vi "Begin.vi"(8 "error in":errorcluster) -> (0 "error out":errorcluster)   [LabVIEW 2019]
doc: "Called before other user functions, this VI is expected to open initial I/O refnums, load in file data, and do all program initialization. Notice that the <B>error out</B> terminal is simply used for data flow. Wiring it to other structures or subVIs ensures that this VI runs first."
uses:
  <vilib>/Rock Robotics/WPI/DriverStation/WPI_DriverStationRobotMode2.ctl
  <vilib>/Rock Robotics/WPI/Joystick/WPI_JoystickDeviceEnum.ctl
  <vilib>/Rock Robotics/WPI/SafetyOutput/WPI_SafetyOutputConfigMenu.ctl
  <vilib>/Rock Robotics/WPI/ThirdParty/Phoenix-LabVIEW/Motor Controller/Controls/CTRE_Phoenix_MotorControl_NeutralMode.ctl
  <vilib>/Rock Robotics/WPI/ThirdParty/Phoenix-LabVIEW/Motor Controller/Controls/CTRE_Phoenix_MotorControl_StatorCurrentLimitConfiguration.ctl
  <vilib>/Rock Robotics/WPI/ThirdParty/Phoenix-LabVIEW/CANCoder/Controls/CTRE_Phoenix_CANcoder_SensorInitializationStrategy.ctl
  <vilib>/Rock Robotics/WPI/ThirdParty/Phoenix-LabVIEW/Motor Controller/Controls/CTRE_Phoenix_MotorControl_FeedbackDevice.ctl
  <vilib>/Rock Robotics/SystemInterfaces/DIO/FPGA_DIOPWMChannel.ctl
  <vilib>/Rock Robotics/WPI/Solenoid/WPI_SolenoidChannel.ctl
  <vilib>/Rock Robotics/SystemInterfaces/DIO/FPGA_DIOChannel.ctl
  Robot Global Data.vi
  <vilib>/Rock Robotics/Network Tables/NT Write String Array.vi
  Refnums.vi
  CAN.vi
  PID.vi
  <vilib>/Rock Robotics/WPI/ThirdParty/Phoenix-LabVIEW/Motor Controller/Sensor/CTRE_Phoenix_MotorControl_SetIntegratedSensorPosition_TalonFX.vi
  <vilib>/Rock Robotics/WPI/RobotDrive/WPI_RobotDriveOpen2MotorWithExistingMotors.vi
  <vilib>/Rock Robotics/WPI/MotorControl/WPI_MotorControlOpen SPARK.vi
  <vilib>/Rock Robotics/WPI/Utilities/WPI_GetSetVariantRefNum.vi
  <vilib>/Rock Robotics/WPI/Solenoid/WPI_SolenoidOpenDouble.vi
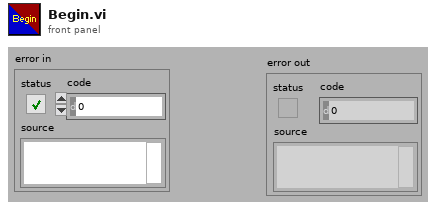
[diagram p1: front panel]
types:
  T1 = typedef "WPI_DriverStationRobotMode2.ctl" = enum16{"Autonomous Disabled", "Autonomous Enabled", "Teleop Disabled", "Teleop Enabled", "Disconnected", "Finish", "Test Disabled", "Test Enabled", "Emergency Stopped"}
  T2 = typedef "WPI_JoystickDeviceEnum.ctl" = enum16{"USB 0", "USB 1", "USB 2", "USB 3", "USB 4", "USB 5"}
  T3 = enum16{"FollowerType_PercentOutput", "FollowerType_AuxOutput1"}
  T4 = typedef "CTRE_Phoenix_CANcoder_SensorInitializationStrategy.ctl" = enum16{"Boot To Zero", "Boot To Absolute Position"}
  T5 = typedef "CTRE_Phoenix_MotorControl_StatorCurrentLimitConfiguration.ctl" = cluster{"Enable?":bool, "Current Limit":dbl, "Threshold Current":dbl, "Threshold Time":dbl}
  T6 = typedef "CTRE_Phoenix_MotorControl_NeutralMode.ctl" = enum8{"EEPROMSetting", "Override to Coast", "Override to Brake"}
  T7 = typedef "WPI_SafetyOutputConfigMenu.ctl" = enum16{"Enable", "Disable"}
  T8 = typedef "FPGA_DIOPWMChannel.ctl" = enum8{"PWM 0", "PWM 1", "PWM 2", "PWM 3", "PWM 4", "PWM 5", "PWM 6", "PWM 7", "PWM 8", "PWM 9", "PWM MXP 0", "PWM MXP 1", "PWM MXP 2", "PWM MXP 3", "PWM MXP 4", "PWM MXP 5", "PWM MXP 6", "PWM MXP 7", "PWM MXP 8", "PWM MXP 9", "Invalid"}
  T9 = enum16{"Blue + Yellow", "Green", "Hot Pink", "Yellow", "Blue", "Red"}
  T10 = typedef "WPI_SolenoidChannel.ctl" = enum8{"Solenoid 0", "Solenoid 1", "Solenoid 2", "Solenoid 3", "Solenoid 4", "Solenoid 5", "Solenoid 6", "Solenoid 7", "Invalid"}
  T11 = typedef "FPGA_DIOChannel.ctl" = enum8{"DIO 0", "DIO 1", "DIO 2", "DIO 3", "DIO 4", "DIO 5", "DIO 6", "DIO 7", "DIO 8", "DIO 9", "DIO MXP 0", "DIO MXP 1", "DIO MXP 2", "DIO MXP 3", "DIO MXP 4", "DIO MXP 5", "DIO MXP 6", "DIO MXP 7", "DIO MXP 8", "DIO MXP 9", "DIO MXP 10", "DIO MXP 11", "DIO MXP 12", "DIO MXP 13", "DIO MXP 14", "DIO MXP 15", "SPI Port CS1", "SPI Port CS2", "SPI Port CS3", "SPI Port MISO", "SPI Port MOSI", "Invalid"}
  T12 = typedef "WPI_JoystickDevRef.ctl" = cluster{"Device":T2}
  T13 = typedef "WPI_MotorControlDeviceRef.ctl" = cluster{"DeviceStatus":errorcluster, "Type":T14, "PWM":cluster{"PWM Channel":T8, "DeadBand":T15}, "CAN":cluster{"Device Number":u8, "SetOutput VI Ref":variant, "GetOutput VI Ref":variant, "Enable VI Ref":variant, "Disable VI Ref":variant, "Data":variant}, "Invert":bool, "DIO PWM":cluster{"PWM \"Enable\" Channel":T8, "DIOChannel":T11, "PWM Rate":dbl}}
  T14 = typedef "WPI_MotorControlType.ctl" = enum16{"PWM", "CAN", "DIO PWM"}
  T15 = typedef "WPI_PWMDeadband.ctl" = cluster{"Name":string, "maxPositivePwm":i32, "minPositivePwm":i32, "centerPwm":i32, "maxNegativePwm":i32, "minNegativePwm":i32, "angularRange":u16}
  T16 = cluster{"P":dbl, "I":dbl, "D":dbl, "F":dbl, "I Zone":dbl}
  T17 = typedef "WPI_RobotDriveDevRef.ctl" = cluster{"DevStatus":errorcluster, "Motors[]":T13[], "Square Inputs":bool, "Max Output":dbl}
  T18 = typedef "CTRE_Phoenix_MotorControl_FeedbackDevice.ctl" = i8
  T19 = typedef "WPI_CompressorDevRef.ctl" = cluster{"DevStatus":errorcluster, "Pneumatics Control Module":u8}
  T20 = typedef "WPI_SolenoidDevRef.ctl" = cluster{"DevStatus":errorcluster, "Pneumatics Control Module":u8, "Forward Solenoid Channel":T10, "Reverse Solenoid Channel":T10}
  T21 = typedef "WPI_DigitalInputDevRef.ctl" = cluster{"DevStatus":errorcluster, "DIO Channel":T11}
  T22 = cluster{"LEFT_MASTER_DRIVE":u8, "RIGHT_FRONT_DRIVE":u8, "RIGHT_MASTER_DRIVE":u8, "RIGHT_REAR_DRIVE":u8, "TURRET":u8, "SHOOTER SLAVE":u8, "SHOOTER":u8, "HOPPER":u8, "LEFT_REAR_DRIVE":u8, "LEFT_FRONT_DRIVE":u8, "INTAKE":u8, "INDEXER":u8, "CLIMBER ARM":u8, "CLIMBER WINCH":u8, "SHOOTER ANGLE":u8, "AGITATOR":u8, "AGITATOR OLD":u8}
  T23 = cluster{"ROBOT_DRIVE":T17, "TURRET":T13, "SHOOTER_MASTER":T13, "HOPPER":T13, "INDEXER":T13, "INTAKE":T13, "CLIMBER_WINCH":T13, "CLIMBER_ARM":T13, "SHOOTER_ANGLE":T13, "SHOOTER_SLAVE":T13, "AGITATOR":T13, "AGITATOR OLD":T13, "LEFT_MASTER":T13, "RIGHT_MASTER":T13}
  T24 = cluster{"COMPRESSOR":T19, "SHIFTER":T20, "INTAKE_PIVOT":T20}
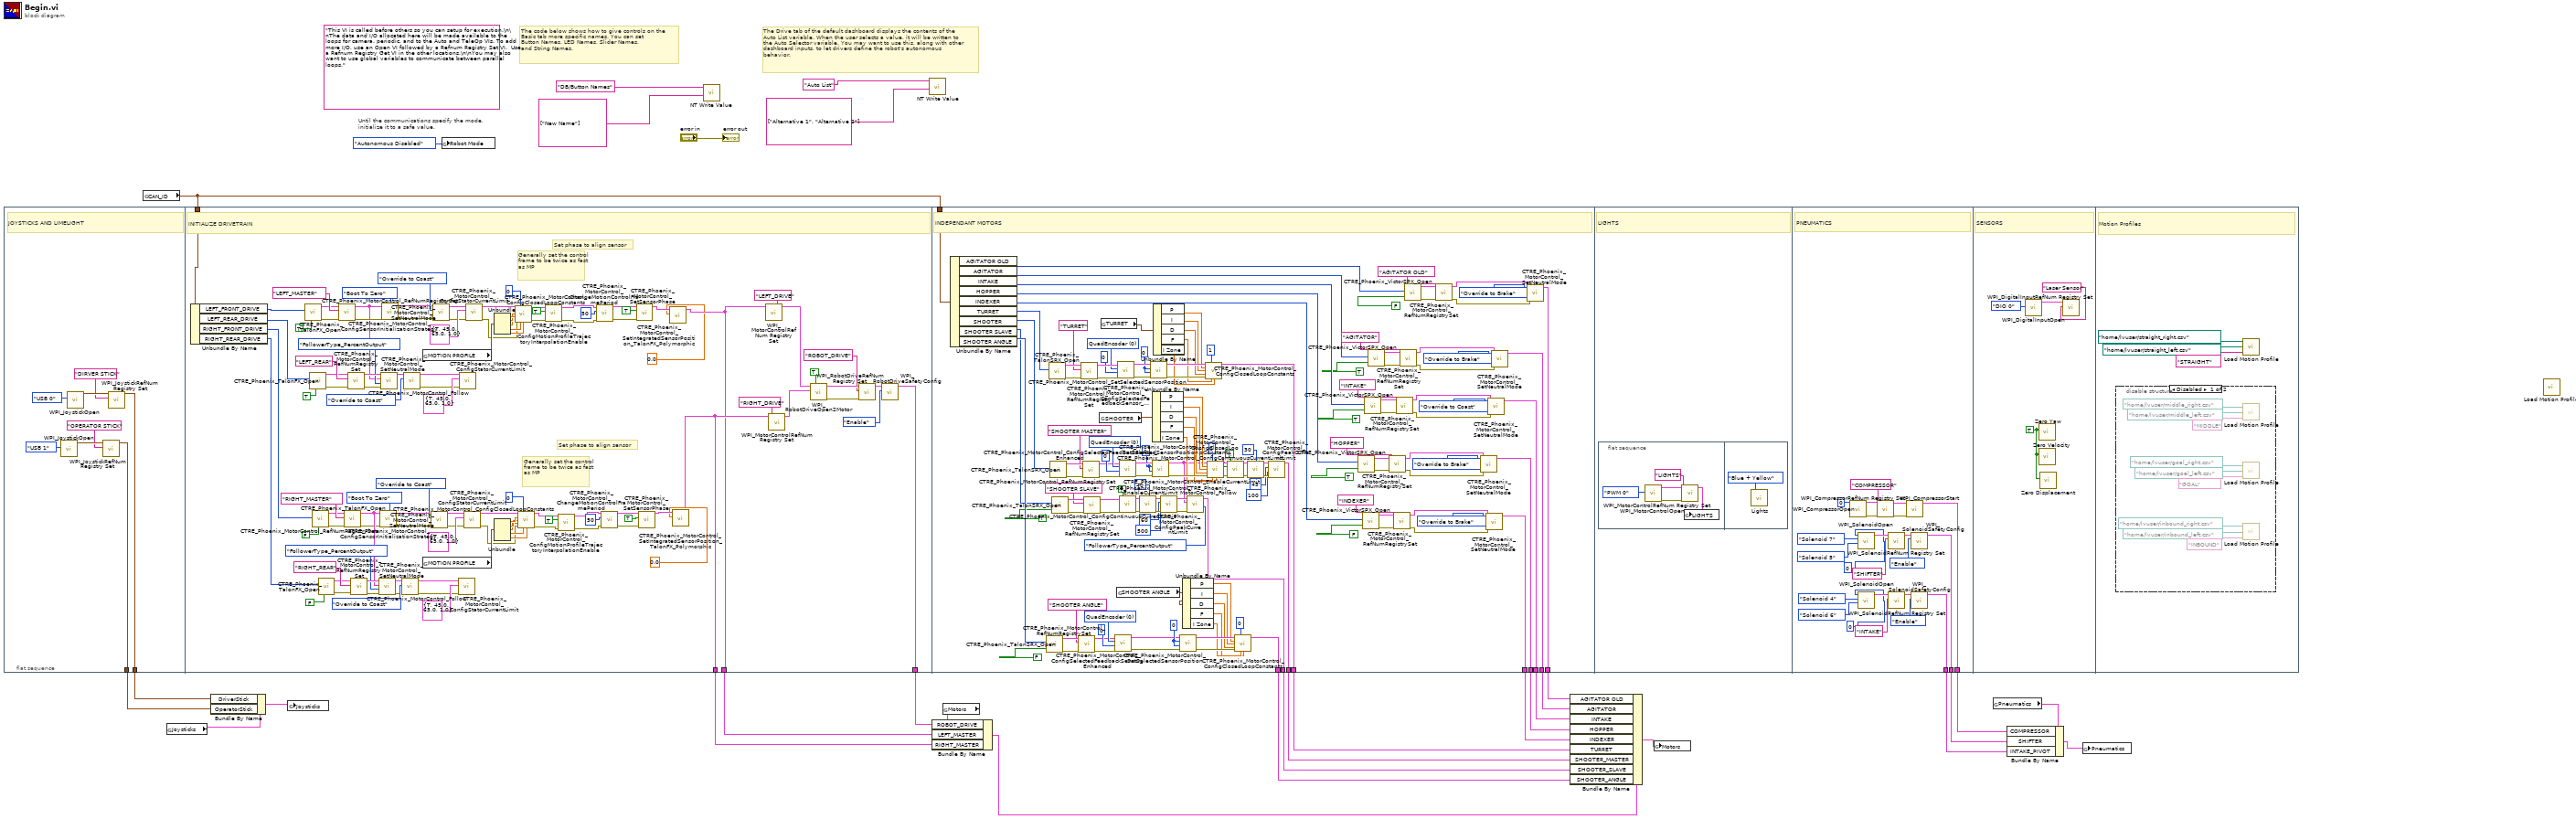
[diagram p0: block diagram]
diagram:
  (unwired) "This VI is called before others so you can setup for execution.\n\nThe data and I/O allocated here will be made available to the loops for camera, periodic, and to the Auto and TeleOp VIs. To add more I/O, use an Open VI followed by a Refnum Registry Set VI.  Use a Refnum Registry Get VI in the other locations.\n\nYou may also want to use global variables to communicate between parallel loops."
  # "The Drive tab of the default dashboard displays the contents of the\nAuto List variable. When the user selects a value, it will be written to\nthe Auto Selector variable. You may want to use this, along with other\ndashboard inputs, to let drivers define the robot's autonomous\nbehavior."
  # "The code below shows how to give controls on the\nBasic tab more specific names. You can set\nButton Names, LED Names, Slider Names,\nand String Names."
  # "Until the communications specify the mode,\ninitialize it to a safe value."
  n1 = flat-sequence {
    tunnel: [w37] -> w24
    tunnel: [w33] -> w14
    tunnel: [w147] -> w20
    tunnel: w22 -> [w146]
    tunnel: [w51] -> w4
    tunnel: [w53] -> w3
    tunnel: [w286] -> w19
    tunnel: w22 -> [w285]
    tunnel: [w208] -> w16
    tunnel: [w284] -> w13
    tunnel: [w188] -> w10
    tunnel: [w171] -> w9
    tunnel: [w170] -> w8
    tunnel: [w169] -> w7
    tunnel: [w160] -> w6
    tunnel: [w148] -> w5
    tunnel: [w309] -> w15
    tunnel: [w302] -> w12
    tunnel: [w295] -> w11
    frame #0 {
      # "JOYSTICKS AND LIMELIGHT"
      n2 = call <vilib>:"WPI_JoystickOpen.vi"("JoystickDevice"=WPI_JoystickDeviceEnum."USB 1") -> ("JoystickDevRef"=w35:T12)  [unwired: 10 in]
      n3 = call <vilib>:"WPI_JoystickOpen.vi"("JoystickDevice"=WPI_JoystickDeviceEnum."USB 0") -> ("JoystickDevRef"=w39:T12)  [unwired: 10 in]
      n4 = call <vilib>:"WPI_JoystickRefNum Registry Set.vi"("refnum name"="OPERATOR STICK", "JoystickDevRef"=w35) -> ("JoystickDevRef"=w33:T12)  [unwired: 8 in, 1 out]
      n5 = call <vilib>:"WPI_JoystickRefNum Registry Set.vi"("refnum name"="DIRVER STICK", "JoystickDevRef"=w39) -> ("JoystickDevRef"=w37:T12)  [unwired: 8 in, 1 out]
    }
    frame #1 {
      # "Set phase to align sensor"
      # "Generally set the control frame to be twice as fast as MP"
      # "Set phase to align sensor"
      # "Generally set the control frame to be twice as fast as MP"
      # "INITIALIZE DRIVETRAIN"
      n6 = Unbundle By Name(w146) -> ("LEFT_FRONT_DRIVE"=w124:u8, "LEFT_REAR_DRIVE"=w120:u8, "RIGHT_FRONT_DRIVE"=w116:u8, "RIGHT_REAR_DRIVE"=w112:u8)
      n7 = call <vilib>:"CTRE_Phoenix_TalonFX_Open.vi"("Invert"=TRUE, "Device Number"=w124) -> ("error out"=w125:errorcluster, "CAN Talon SRX Ref"=w126:T13)  [unwired: 8 in]
      n8 = call <vilib>:"CTRE_Phoenix_TalonFX_Open.vi"("Invert"=TRUE, "Device Number"=w120) -> ("error out"=w122:errorcluster, "CAN Talon SRX Ref"=w123:T13)  [unwired: 8 in]
      n9 = call <vilib>:"CTRE_Phoenix_TalonFX_Open.vi"("Invert"=FALSE, "Device Number"=w116) -> ("error out"=w119:errorcluster, "CAN Talon SRX Ref"=w118:T13)  [unwired: 8 in]
      n10 = call <vilib>:"CTRE_Phoenix_TalonFX_Open.vi"("Invert"=FALSE, "Device Number"=w112) -> ("error out"=w113:errorcluster, "CAN Talon SRX Ref"=w114:T13)  [unwired: 8 in]
      n11 = call <vilib>:"CTRE_Phoenix_MotorControl_RefNumRegistrySet.vi"("error in (no error)"=w125, "refnum name"="LEFT_MASTER", "PhoenixMotorControlDevRef"=w126) -> ("error out"=w107:errorcluster, "PhoenixMotorControlDevRef"=w88:T13)  [unwired: 7 in]
      n12 = call <vilib>:"CTRE_Phoenix_MotorControl_RefNumRegistrySet.vi"("error in (no error)"=w119, "refnum name"="RIGHT_MASTER", "PhoenixMotorControlDevRef"=w118) -> ("error out"=w60:errorcluster, "PhoenixMotorControlDevRef"=w89:T13)  [unwired: 7 in]
      n13 = call <vilib>:"CTRE_Phoenix_MotorControl_RefNumRegistrySet.vi"("error in (no error)"=w122, "refnum name"="LEFT_REAR", "PhoenixMotorControlDevRef"=w123) -> ("error out"=w143:errorcluster, "PhoenixMotorControlDevRef"=w144:T13)  [unwired: 7 in]
      n14 = call <vilib>:"CTRE_Phoenix_MotorControl_RefNumRegistrySet.vi"("error in (no error)"=w113, "refnum name"="RIGHT_REAR", "PhoenixMotorControlDevRef"=w114) -> ("error out"=w90:errorcluster, "PhoenixMotorControlDevRef"=w91:T13)  [unwired: 7 in]
      n15 = call <vilib>:"CTRE_Phoenix_MotorControl_Follow.vi"("error in (no error)"=w90, "FollowerType"=T3."FollowerType_PercentOutput", "Master Controller to Follow"=w89, "PhoenixMotorControlDevRef"=w91) -> ("error out"=w87:errorcluster, "PhoenixMotorControlDevRef"=w101:T13)  [unwired: 6 in]
      n16 = call <vilib>:"CTRE_Phoenix_MotorControl_ConfigSensorInitializationStrategy.vi"("error in (no error)"=w60, "Sensor Initialization Strategy"=CTRE_Phoenix_CANcoder_SensorInitializationStrategy."Boot To Zero", "PhoenixMotorControlDevRef"=w89) -> ("error out"=w94:errorcluster, "PhoenixMotorControlDevRef"=w95:T13)  [unwired: 7 in]
      n17 = call <vilib>:"CTRE_Phoenix_MotorControl_Follow.vi"("error in (no error)"=w143, "FollowerType"=T3."FollowerType_PercentOutput", "Master Controller to Follow"=w88, "PhoenixMotorControlDevRef"=w144) -> ("PhoenixMotorControlDevRef"=w130:T13)  [unwired: 6 in, 1 out]
      n18 = call <vilib>:"CTRE_Phoenix_MotorControl_ConfigSensorInitializationStrategy.vi"("error in (no error)"=w107, "Sensor Initialization Strategy"=CTRE_Phoenix_CANcoder_SensorInitializationStrategy."Boot To Zero", "PhoenixMotorControlDevRef"=w88) -> ("error out"=w105:errorcluster, "PhoenixMotorControlDevRef"=w106:T13)  [unwired: 7 in]
      n19 = call <vilib>:"CTRE_Phoenix_MotorControl_SetNeutralMode.vi"("error in (no error)"=w87, "Motor Control Neutral Mode"=CTRE_Phoenix_MotorControl_NeutralMode."Override to Coast", "PhoenixMotorControlDevRef"=w101) -> ("error out"=w92:errorcluster, "PhoenixMotorControlDevRef"=w93:T13)  [unwired: 7 in]
      n20 = call <vilib>:"CTRE_Phoenix_MotorControl_SetNeutralMode.vi"("Motor Control Neutral Mode"=CTRE_Phoenix_MotorControl_NeutralMode."Override to Coast", "PhoenixMotorControlDevRef"=w130) -> ("error out"=w103:errorcluster, "PhoenixMotorControlDevRef"=w104:T13)  [unwired: 8 in]
      n21 = global read "PID.vi" "MOTION PROFILE"() -> (w83:T16)
      n22 = global read "PID.vi" "MOTION PROFILE"() -> (w77:T16)
      n23 = call <vilib>:"CTRE_Phoenix_MotorControl_SetNeutralMode.vi"("error in (no error)"=w94, "Motor Control Neutral Mode"=CTRE_Phoenix_MotorControl_NeutralMode."Override to Coast", "PhoenixMotorControlDevRef"=w95) -> ("error out"=w59:errorcluster, "PhoenixMotorControlDevRef"=w97:T13)  [unwired: 7 in]
      n24 = call <vilib>:"CTRE_Phoenix_MotorControl_SetNeutralMode.vi"("error in (no error)"=w105, "Motor Control Neutral Mode"=CTRE_Phoenix_MotorControl_NeutralMode."Override to Coast", "PhoenixMotorControlDevRef"=w106) -> ("error out"=w57:errorcluster, "PhoenixMotorControlDevRef"=w109:T13)  [unwired: 7 in]
      n25 = call <vilib>:"CTRE_Phoenix_MotorControl_ConfigStatorCurrentLimit.vi"("error in (no error)"=w92, "Stator Current Limit Configuration"=T5 {"Enable?"=TRUE, "Current Limit"=45.0, "Threshold Current"=65.0, "Threshold Time"=1.0}, "PhoenixMotorControlDevRef"=w93) -> ()  [unwired: 7 in, 2 out]
      n26 = call <vilib>:"CTRE_Phoenix_MotorControl_ConfigStatorCurrentLimit.vi"("error in (no error)"=w103, "Stator Current Limit Configuration"=T5 {"Enable?"=TRUE, "Current Limit"=45.0, "Threshold Current"=65.0, "Threshold Time"=1.0}, "PhoenixMotorControlDevRef"=w104) -> ()  [unwired: 7 in, 2 out]
      n27 = call <vilib>:"CTRE_Phoenix_MotorControl_ConfigStatorCurrentLimit.vi"("error in (no error)"=w59, "Stator Current Limit Configuration"=T5 {"Enable?"=TRUE, "Current Limit"=45.0, "Threshold Current"=65.0, "Threshold Time"=1.0}, "PhoenixMotorControlDevRef"=w97) -> ("error out"=w58:errorcluster, "PhoenixMotorControlDevRef"=w71:T13)  [unwired: 7 in]
      n28 = call <vilib>:"CTRE_Phoenix_MotorControl_ConfigStatorCurrentLimit.vi"("error in (no error)"=w57, "Stator Current Limit Configuration"=T5 {"Enable?"=TRUE, "Current Limit"=45.0, "Threshold Current"=65.0, "Threshold Time"=1.0}, "PhoenixMotorControlDevRef"=w109) -> ("error out"=w56:errorcluster, "PhoenixMotorControlDevRef"=w84:T13)  [unwired: 7 in]
      n29 = Unbundle(w83) -> ("P"=w82:dbl, "I"=w81:dbl, "D"=w80:dbl, "F"=w79:dbl, "I Zone"=w78:dbl)
      n30 = Unbundle(w77) -> ("P"=w76:dbl, "I"=w75:dbl, "D"=w74:dbl, "F"=w73:dbl, "I Zone"=w72:dbl)
      n31 = call <vilib>:"CTRE_Phoenix_MotorControl_ConfigClosedLoopConstants.vi"("PhoenixMotorControlDevRef"=w84, "slotIdx"=0, "P"=w82, "I"=w81, "D"=w80, "error in (no error)"=w56, "F"=w79, "I Zone"=w78) -> ("PhoenixMotorControlDevRef"=w44:T13, "error out"=w41:errorcluster)  [unwired: 6 in]
      n32 = call <vilib>:"CTRE_Phoenix_MotorControl_ConfigClosedLoopConstants.vi"("PhoenixMotorControlDevRef"=w71, "slotIdx"=0, "P"=w76, "I"=w75, "D"=w74, "error in (no error)"=w58, "F"=w73, "I Zone"=w72) -> ("PhoenixMotorControlDevRef"=w49:T13, "error out"=w47:errorcluster)  [unwired: 6 in]
      n33 = call <vilib>:"CTRE_Phoenix_MotorControl_ConfigMotionProfileTrajectoryInterpolationEnable.vi"("error in"=w41, "enable?"=TRUE, "PhoenixMotorControlDevRef"=w44) -> ("error out"=w40:errorcluster, "PhoenixMotorControlDevRef"=w43:T13)  [unwired: 7 in]
      n34 = call <vilib>:"CTRE_Phoenix_MotorControl_ConfigMotionProfileTrajectoryInterpolationEnable.vi"("error in"=w47, "enable?"=TRUE, "PhoenixMotorControlDevRef"=w49) -> ("error out"=w45:errorcluster, "PhoenixMotorControlDevRef"=w46:T13)  [unwired: 7 in]
      n35 = call <vilib>:"CTRE_Phoenix_MotorControl_ChangeMotionControlFramePeriod.vi"("error in"=w40, "periodMs"=50, "PhoenixMotorControlDevRef"=w43) -> ("error out"=w65:errorcluster, "PhoenixMotorControlDevRef"=w66:T13)  [unwired: 7 in]
      n36 = call <vilib>:"CTRE_Phoenix_MotorControl_ChangeMotionControlFramePeriod.vi"("error in"=w45, "periodMs"=50, "PhoenixMotorControlDevRef"=w46) -> ("error out"=w61:errorcluster, "PhoenixMotorControlDevRef"=w62:T13)  [unwired: 7 in]
      n37 = call <vilib>:"CTRE_Phoenix_MotorControl_SetSensorPhase.vi"("error in (no error)"=w65, "PhaseSensor"=TRUE, "PhoenixMotorControlDevRef"=w66) -> ("PhoenixMotorControlDevRef"=w52:T13)  [unwired: 7 in, 1 out]
      n38 = call <vilib>:"CTRE_Phoenix_MotorControl_SetSensorPhase.vi"("error in (no error)"=w61, "PhaseSensor"=TRUE, "PhoenixMotorControlDevRef"=w62) -> ("PhoenixMotorControlDevRef"=w55:T13)  [unwired: 7 in, 1 out]
      n39 = call-poly <vilib>:"CTRE_Phoenix_MotorControl_SetIntegratedSensorPosition_TalonFX_Polymorphic.vi"("New Position"=0.0, "PhoenixMotorControlDevRef"=w52) -> ("PhoenixMotorControlDevRef"=w51:T13)  [unwired: 8 in, 1 out]
      n40 = call-poly <vilib>:"CTRE_Phoenix_MotorControl_SetIntegratedSensorPosition_TalonFX_Polymorphic.vi"("New Position"=0.0, "PhoenixMotorControlDevRef"=w55) -> ("PhoenixMotorControlDevRef"=w53:T13)  [unwired: 8 in, 1 out]
      n41 = call <vilib>:"WPI_MotorControlRefNum Registry Set.vi"("refnum name"="LEFT_DRIVE", "MotorControlDevRef"=w51) -> ()  [unwired: 8 in, 2 out]
      n42 = call <vilib>:"WPI_MotorControlRefNum Registry Set.vi"("refnum name"="RIGHT_DRIVE", "MotorControlDevRef"=w53) -> ("MotorControlDevRef"=w145:T13)  [unwired: 8 in, 1 out]
      n43 = call-poly <vilib>:"WPI_RobotDriveOpen2Motor.vi"("Square Inputs"=TRUE, "Right Motor Dev Ref"=w145, "Left Motor Dev Ref"=w51) -> ("error out"=w136:errorcluster, "RobotDriveDevRef"=w135:T17)  [unwired: 2 in, 5 out]
      n44 = call <vilib>:"WPI_RobotDriveRefNum Registry Set.vi"("error in (no error)"=w136, "refnum name"="ROBOT_DRIVE", "RobotDriveDevRef"=w135) -> ("RobotDriveDevRef"=w134:T17)  [unwired: 1 in, 7 out]
      n45 = call <vilib>:"WPI_RobotDriveSafetyConfig.vi"("mode"=WPI_SafetyOutputConfigMenu."Enable", "RobotDriveDevRef"=w134) -> ("RobotDriveDevRef"=w147:T17)  [unwired: 8 in, 1 out]
    }
    frame #2 {
      w242 = 0 ("New Sensor Position")
      w244 = T18 0 items=["QuadEncoder"=0, "Analog"=2, "Tachometer"=4, "Pulse Width Encoded Position"=8, "Sensor Sum (S0 + S1)"=9, "Sensor Difference (D0 - D1)"=10, "Remote Source 0"=11, "Remote Source 1"=12, "Software Emulated"=15] ("Feedback Device")
      w184 = 0 ("New Sensor Position")
      w261 = T18 0 items=["QuadEncoder"=0, "Analog"=2, "Tachometer"=4, "Pulse Width Encoded Position"=8, "Sensor Sum (S0 + S1)"=9, "Sensor Difference (D0 - D1)"=10, "Remote Source 0"=11, "Remote Source 1"=12, "Software Emulated"=15] ("Feedback Device")
      w274 = 0 ("New Sensor Position")
      w278 = T18 0 items=["QuadEncoder"=0, "Analog"=2, "Tachometer"=4, "Pulse Width Encoded Position"=8, "Sensor Sum (S0 + S1)"=9, "Sensor Difference (D0 - D1)"=10, "Remote Source 0"=11, "Remote Source 1"=12, "Software Emulated"=15] ("Feedback Device")
      # "INDEPENDANT MOTORS"
      n46 = Unbundle By Name(w285) -> ("AGITATOR OLD"=w149:u8, "AGITATOR"=w161:u8, "INTAKE"=w174:u8, "HOPPER"=w173:u8, "INDEXER"=w172:u8, "TURRET"=w265:u8, "SHOOTER"=w249:u8, "SHOOTER SLAVE"=w187:u8, "SHOOTER ANGLE"=w230:u8)
      n47 = call <vilib>:"CTRE_Phoenix_TalonSRX_Open.vi"("Invert"=FALSE, "Device Number"=w230) -> ("error out"=w247:errorcluster, "CAN Talon SRX Ref"=w246:T13)  [unwired: 8 in]
      n48 = call <vilib>:"CTRE_Phoenix_TalonSRX_Open.vi"("Device Number"=w265) -> ("error out"=w283:errorcluster, "CAN Talon SRX Ref"=w282:T13)  [unwired: 9 in]
      n49 = call <vilib>:"CTRE_Phoenix_TalonSRX_Open.vi"("Device Number"=w249) -> ("error out"=w264:errorcluster, "CAN Talon SRX Ref"=w263:T13)  [unwired: 9 in]
      n50 = call <vilib>:"CTRE_Phoenix_TalonSRX_Open.vi"("Invert"=TRUE, "Device Number"=w187) -> ("error out"=w205:errorcluster, "CAN Talon SRX Ref"=w204:T13)  [unwired: 8 in]
      n51 = call <vilib>:"CTRE_Phoenix_MotorControl_RefNumRegistrySet.vi"("error in (no error)"=w247, "refnum name"="SHOOTER ANGLE", "PhoenixMotorControlDevRef"=w246) -> ("error out"=w245:errorcluster, "PhoenixMotorControlDevRef"=w232:T13)  [unwired: 7 in]
      n52 = call <vilib>:"CTRE_Phoenix_MotorControl_RefNumRegistrySet.vi"("error in (no error)"=w283, "refnum name"="TURRET", "PhoenixMotorControlDevRef"=w282) -> ("error out"=w280:errorcluster, "PhoenixMotorControlDevRef"=w279:T13)  [unwired: 7 in]
      n53 = call <vilib>:"CTRE_Phoenix_MotorControl_RefNumRegistrySet.vi"("error in (no error)"=w264, "refnum name"="SHOOTER MASTER", "PhoenixMotorControlDevRef"=w263) -> ("error out"=w262:errorcluster, "PhoenixMotorControlDevRef"=w223:T13)  [unwired: 7 in]
      n54 = call <vilib>:"CTRE_Phoenix_MotorControl_RefNumRegistrySet.vi"("error in (no error)"=w205, "refnum name"="SHOOTER SLAVE", "PhoenixMotorControlDevRef"=w204) -> ("error out"=w193:errorcluster, "PhoenixMotorControlDevRef"=w194:T13)  [unwired: 7 in]
      n55 = global read "PID.vi" "SHOOTER"() -> (w256:T16)
      n56 = global read "PID.vi" "TURRET"() -> (w271:T16)
      n57 = call <vilib>:"CTRE_Phoenix_MotorControl_ConfigSelectedFeedbackSensor_Enhanced.vi"("error in (no error)"=w245, "pidLoopIdx"=0, "Feedback Device"=w244, "PhoenixMotorControlDevRef"=w232) -> ("error out"=w157:errorcluster, "PhoenixMotorControlDevRef"=w158:T13)  [unwired: 6 in]
      n58 = global read "PID.vi" "SHOOTER ANGLE"() -> (w239:T16)
      n59 = call <vilib>:"CTRE_Phoenix_MotorControl_ConfigSelectedFeedbackSensor_Enhanced.vi"("error in (no error)"=w280, "pidLoopIdx"=0, "Feedback Device"=w278, "PhoenixMotorControlDevRef"=w279) -> ("error out"=w276:errorcluster, "PhoenixMotorControlDevRef"=w275:T13)  [unwired: 6 in]
      n60 = call <vilib>:"CTRE_Phoenix_MotorControl_ConfigSelectedFeedbackSensor_Enhanced.vi"("error in (no error)"=w262, "pidLoopIdx"=0, "Feedback Device"=w261, "PhoenixMotorControlDevRef"=w223) -> ("error out"=w259:errorcluster, "PhoenixMotorControlDevRef"=w258:T13)  [unwired: 6 in]
      n61 = call <vilib>:"CTRE_Phoenix_MotorControl_EnableCurrentLimit.vi"("error in (no error)"=w193, "Enable Current Limit?"=TRUE, "PhoenixMotorControlDevRef"=w194) -> ("error out"=w201:errorcluster, "PhoenixMotorControlDevRef"=w200:T13)  [unwired: 7 in]
      n62 = call <vilib>:"CTRE_Phoenix_MotorControl_ConfigContinuousCurrentLimit.vi"("error in (no error)"=w201, "Continuous Current Limit (Amps)"=40, "PhoenixMotorControlDevRef"=w200) -> ("error out"=w198:errorcluster, "PhoenixMotorControlDevRef"=w197:T13)  [unwired: 7 in]
      n63 = call <vilib>:"CTRE_Phoenix_MotorControl_SetSelectedSensorPosition.vi"("error in (no error)"=w276, "pidLoopIdx"=w274, "New Sensor Position"=w274, "PhoenixMotorControlDevRef"=w275) -> ("error out"=w272:errorcluster, "PhoenixMotorControlDevRef"=w273:T13)  [unwired: 6 in]
      n64 = Unbundle By Name(w256) -> ("P"=w250:dbl, "I"=w255:dbl, "D"=w254:dbl, "F"=w253:dbl, "I Zone"=w252:dbl)
      n65 = call <vilib>:"CTRE_Phoenix_MotorControl_SetSelectedSensorPosition.vi"("error in (no error)"=w259, "pidLoopIdx"=w184, "New Sensor Position"=w184, "PhoenixMotorControlDevRef"=w258) -> ("error out"=w257:errorcluster, "PhoenixMotorControlDevRef"=w190:T13)  [unwired: 6 in]
      n66 = Unbundle By Name(w271) -> ("P"=w270:dbl, "I"=w269:dbl, "D"=w268:dbl, "F"=w185:dbl, "I Zone"=w267:dbl)
      n67 = call <vilib>:"CTRE_Phoenix_MotorControl_ConfigPeakCurrentLimit.vi"("error in (no error)"=w198, "Peak Current Maximum Duration (ms)"=500, "Peak Current (Amps)"=60, "PhoenixMotorControlDevRef"=w197) -> ("error out"=w192:errorcluster, "PhoenixMotorControlDevRef"=w191:T13)  [unwired: 6 in]
      n68 = call <vilib>:"CTRE_Phoenix_MotorControl_SetSelectedSensorPosition.vi"("error in (no error)"=w157, "pidLoopIdx"=w242, "New Sensor Position"=w242, "PhoenixMotorControlDevRef"=w158) -> ("error out"=w240:errorcluster, "PhoenixMotorControlDevRef"=w241:T13)  [unwired: 6 in]
      n69 = Unbundle By Name(w239) -> ("P"=w233:dbl, "I"=w238:dbl, "D"=w237:dbl, "F"=w236:dbl, "I Zone"=w235:dbl)
      n70 = call <vilib>:"CTRE_Phoenix_MotorControl_Follow.vi"("error in (no error)"=w192, "FollowerType"=T3."FollowerType_PercentOutput", "Master Controller to Follow"=w190, "PhoenixMotorControlDevRef"=w191) -> ("PhoenixMotorControlDevRef"=w188:T13)  [unwired: 6 in, 1 out]
      n71 = call <vilib>:"CTRE_Phoenix_MotorControl_ConfigClosedLoopConstants.vi"("PhoenixMotorControlDevRef"=w273, "slotIdx"=1, "P"=w270, "I"=w269, "D"=w268, "error in (no error)"=w272, "F"=w185, "I Zone"=w267) -> ("PhoenixMotorControlDevRef"=w286:T13)  [unwired: 6 in, 1 out]
      n72 = call <vilib>:"CTRE_Phoenix_MotorControl_ConfigClosedLoopConstants.vi"("PhoenixMotorControlDevRef"=w190, "slotIdx"=0, "P"=w250, "I"=w255, "D"=w254, "error in (no error)"=w257, "F"=w253, "I Zone"=w252) -> ("PhoenixMotorControlDevRef"=w216:T13, "error out"=w214:errorcluster)  [unwired: 6 in]
      n73 = call <vilib>:"CTRE_Phoenix_MotorControl_EnableCurrentLimit.vi"("error in (no error)"=w214, "Enable Current Limit?"=TRUE, "PhoenixMotorControlDevRef"=w216) -> ("error out"=w213:errorcluster, "PhoenixMotorControlDevRef"=w212:T13)  [unwired: 7 in]
      n74 = call <vilib>:"CTRE_Phoenix_MotorControl_ConfigClosedLoopConstants.vi"("PhoenixMotorControlDevRef"=w241, "slotIdx"=0, "P"=w233, "I"=w238, "D"=w237, "error in (no error)"=w240, "F"=w236, "I Zone"=w235) -> ("PhoenixMotorControlDevRef"=w284:T13)  [unwired: 6 in, 1 out]
      n75 = call <vilib>:"CTRE_Phoenix_MotorControl_ConfigContinuousCurrentLimit.vi"("error in (no error)"=w213, "Continuous Current Limit (Amps)"=30, "PhoenixMotorControlDevRef"=w212) -> ("error out"=w210:errorcluster, "PhoenixMotorControlDevRef"=w209:T13)  [unwired: 7 in]
      n76 = call <vilib>:"CTRE_Phoenix_MotorControl_ConfigPeakCurrentLimit.vi"("error in (no error)"=w210, "Peak Current Maximum Duration (ms)"=100, "Peak Current (Amps)"=45, "PhoenixMotorControlDevRef"=w209) -> ("PhoenixMotorControlDevRef"=w208:T13)  [unwired: 6 in, 1 out]
      n77 = call <vilib>:"CTRE_Phoenix_VictorSPX_Open.vi"("Invert"=TRUE, "Device Number"=w173) -> ("error out"=w222:errorcluster, "CAN Talon SRX Ref"=w221:T13)  [unwired: 8 in]
      n78 = call <vilib>:"CTRE_Phoenix_VictorSPX_Open.vi"("Invert"=FALSE, "Device Number"=w172) -> ("error out"=w181:errorcluster, "CAN Talon SRX Ref"=w180:T13)  [unwired: 8 in]
      n79 = call <vilib>:"CTRE_Phoenix_VictorSPX_Open.vi"("Invert"=TRUE, "Device Number"=w174) -> ("error out"=w229:errorcluster, "CAN Talon SRX Ref"=w228:T13)  [unwired: 8 in]
      n80 = call <vilib>:"CTRE_Phoenix_VictorSPX_Open.vi"("Invert"=TRUE, "Device Number"=w161) -> ("error out"=w168:errorcluster, "CAN Talon SRX Ref"=w167:T13)  [unwired: 8 in]
      n81 = call <vilib>:"CTRE_Phoenix_MotorControl_RefNumRegistrySet.vi"("error in (no error)"=w222, "refnum name"="HOPPER", "PhoenixMotorControlDevRef"=w221) -> ("error out"=w219:errorcluster, "PhoenixMotorControlDevRef"=w218:T13)  [unwired: 7 in]
      n82 = call <vilib>:"CTRE_Phoenix_MotorControl_RefNumRegistrySet.vi"("error in (no error)"=w181, "refnum name"="INDEXER", "PhoenixMotorControlDevRef"=w180) -> ("error out"=w178:errorcluster, "PhoenixMotorControlDevRef"=w177:T13)  [unwired: 7 in]
      n83 = call <vilib>:"CTRE_Phoenix_MotorControl_RefNumRegistrySet.vi"("error in (no error)"=w229, "refnum name"="INTAKE", "PhoenixMotorControlDevRef"=w228) -> ("error out"=w226:errorcluster, "PhoenixMotorControlDevRef"=w225:T13)  [unwired: 7 in]
      n84 = call <vilib>:"CTRE_Phoenix_MotorControl_RefNumRegistrySet.vi"("error in (no error)"=w168, "refnum name"="AGITATOR", "PhoenixMotorControlDevRef"=w167) -> ("error out"=w165:errorcluster, "PhoenixMotorControlDevRef"=w164:T13)  [unwired: 7 in]
      n85 = call <vilib>:"CTRE_Phoenix_VictorSPX_Open.vi"("Invert"=FALSE, "Device Number"=w149) -> ("error out"=w156:errorcluster, "CAN Talon SRX Ref"=w155:T13)  [unwired: 8 in]
      n86 = call <vilib>:"CTRE_Phoenix_MotorControl_RefNumRegistrySet.vi"("error in (no error)"=w156, "refnum name"="AGITATOR OLD", "PhoenixMotorControlDevRef"=w155) -> ("error out"=w153:errorcluster, "PhoenixMotorControlDevRef"=w152:T13)  [unwired: 7 in]
      n87 = call <vilib>:"CTRE_Phoenix_MotorControl_SetNeutralMode.vi"("error in (no error)"=w219, "Motor Control Neutral Mode"=CTRE_Phoenix_MotorControl_NeutralMode."Override to Brake", "PhoenixMotorControlDevRef"=w218) -> ("PhoenixMotorControlDevRef"=w170:T13)  [unwired: 7 in, 1 out]
      n88 = call <vilib>:"CTRE_Phoenix_MotorControl_SetNeutralMode.vi"("error in (no error)"=w178, "Motor Control Neutral Mode"=CTRE_Phoenix_MotorControl_NeutralMode."Override to Brake", "PhoenixMotorControlDevRef"=w177) -> ("PhoenixMotorControlDevRef"=w169:T13)  [unwired: 7 in, 1 out]
      n89 = call <vilib>:"CTRE_Phoenix_MotorControl_SetNeutralMode.vi"("error in (no error)"=w226, "Motor Control Neutral Mode"=CTRE_Phoenix_MotorControl_NeutralMode."Override to Coast", "PhoenixMotorControlDevRef"=w225) -> ("PhoenixMotorControlDevRef"=w171:T13)  [unwired: 7 in, 1 out]
      n90 = call <vilib>:"CTRE_Phoenix_MotorControl_SetNeutralMode.vi"("error in (no error)"=w165, "Motor Control Neutral Mode"=CTRE_Phoenix_MotorControl_NeutralMode."Override to Brake", "PhoenixMotorControlDevRef"=w164) -> ("PhoenixMotorControlDevRef"=w160:T13)  [unwired: 7 in, 1 out]
      n91 = call <vilib>:"CTRE_Phoenix_MotorControl_SetNeutralMode.vi"("error in (no error)"=w153, "Motor Control Neutral Mode"=CTRE_Phoenix_MotorControl_NeutralMode."Override to Brake", "PhoenixMotorControlDevRef"=w152) -> ("PhoenixMotorControlDevRef"=w148:T13)  [unwired: 7 in, 1 out]
    }
    frame #3 {
      # "LIGHTS"
      n92 = flat-sequence {
        frame #0 {
          n93 = call-poly <vilib>:"WPI_MotorControlOpen.vi"("PWM Channel"=FPGA_DIOPWMChannel."PWM 0") -> ("error out"=w290:errorcluster, "MotorControlDeviceRef"=w291:T13)  [unwired: 9 in]
          n94 = call <vilib>:"WPI_MotorControlRefNum Registry Set.vi"("error in (no error)"=w290, "refnum name"="LIGHTS", "MotorControlDevRef"=w291) -> ("MotorControlDevRef"=w287:T13)  [unwired: 7 in, 1 out]
          n95 = global write "Refnums.vi" "LIGHTS"(w287) -> ()
        }
        frame #1 {
          n96 = call "Lights.vi"("Colour"=T9."Blue + Yellow") -> ()  [unwired: 11 in]
        }
      }
    }
    frame #4 {
      # "PNEUMATICS"
      n97 = call <vilib>:"WPI_CompressorOpen.vi"("Pneumatics Control Module (0)"=u8 0) -> ("CompressorDevRef"=w313:T19, "error out"=w314:errorcluster)  [unwired: 13 in]
      n98 = call-poly <vilib>:"WPI_SolenoidOpen.vi"("Reverse Solenoid Channel"=WPI_SolenoidChannel."Solenoid 5", "Forward Solenoid Channel"=WPI_SolenoidChannel."Solenoid 7", "Pneumatics Control Module (0)"=u8 0) -> ("SolenoidDevRef"=w308:T20)  [unwired: 7 in, 1 out]
      n99 = call-poly <vilib>:"WPI_SolenoidOpen.vi"("Reverse Solenoid Channel"=WPI_SolenoidChannel."Solenoid 6", "Forward Solenoid Channel"=WPI_SolenoidChannel."Solenoid 4", "Pneumatics Control Module (0)"=u8 0) -> ("SolenoidDevRef"=w301:T20)  [unwired: 7 in, 1 out]
      n100 = call <vilib>:"WPI_CompressorRefNum Registry Set.vi"("error in (no error)"=w314, "refnum name"="COMPRESSOR", "CompressorDevRef"=w313) -> ("error out"=w311:errorcluster, "CompressorDevRef"=w310:T19)  [unwired: 7 in]
      n101 = call <vilib>:"WPI_SolenoidRefNum Registry Set.vi"("refnum name"="SHIFTER", "SolenoidDevRef"=w308) -> ("SolenoidDevRef"=w304:T20)  [unwired: 8 in, 1 out]
      n102 = call <vilib>:"WPI_SolenoidRefNum Registry Set.vi"("refnum name"="INTAKE", "SolenoidDevRef"=w301) -> ("SolenoidDevRef"=w297:T20)  [unwired: 8 in, 1 out]
      n103 = call <vilib>:"WPI_CompressorStart.vi"("error in (no error)"=w311, "CompressorDevRef"=w310) -> ("CompressorDevRef"=w309:T19)  [unwired: 8 in, 1 out]
      n104 = call <vilib>:"WPI_SolenoidSafetyConfig.vi"("mode"=WPI_SafetyOutputConfigMenu."Enable", "SolenoidDevRef"=w304) -> ("SolenoidDevRef"=w302:T20)  [unwired: 8 in, 1 out]
      n105 = call <vilib>:"WPI_SolenoidSafetyConfig.vi"("mode"=WPI_SafetyOutputConfigMenu."Enable", "SolenoidDevRef"=w297) -> ("SolenoidDevRef"=w295:T20)  [unwired: 8 in, 1 out]
    }
    frame #5 {
      w316 = TRUE ("Zero")
      # "SENSORS"
      n106 = call <vilib>:"WPI_DigitalInputOpen.vi"("DIO Channel"=FPGA_DIOChannel."DIO 0") -> ("DigitalInputDevRef"=w317:T21)  [unwired: 9 in, 1 out]
      n107 = call <vilib>:"Zero Yaw.vi"("Zero"=w316) -> ()  [unwired: 11 in]
      n108 = call <vilib>:"Zero Velocity.vi"("Zero"=w316) -> ()  [unwired: 11 in]
      n109 = call <vilib>:"Zero Displacement.vi"("Zero"=w316) -> ()  [unwired: 11 in]
      n110 = call <vilib>:"WPI_DigitalInputRefNum Registry Set.vi"("refnum name"="Laser Sensor", "DigitalInputDevRef"=w317) -> ()  [unwired: 8 in, 2 out]
    }
    frame #6 {
      # "Motion Profiles"
      n111 = disable-structure shown="Disabled" {
        frame Disabled {
          n112 = call "Load Motion Profile.vi"("Refnum Name"="MIDDLE", "Left File Path"=path "/home/lvuser/middle_left.csv", "Right File Path"=path "/home/lvuser/middle_right.csv") -> ()  [unwired: 2 in]
          n113 = call "Load Motion Profile.vi"("Refnum Name"="GOAL", "Left File Path"=path "/home/lvuser/goal_left.csv", "Right File Path"=path "/home/lvuser/goal_right.csv") -> ()  [unwired: 2 in]
          n114 = call "Load Motion Profile.vi"("Refnum Name"="INBOUND", "Left File Path"=path "/home/lvuser/inbound_left.csv", "Right File Path"=path "/home/lvuser/inbound_right.csv") -> ()  [unwired: 2 in]
        }
        frame Enabled {
        }
      }
      n115 = call "Load Motion Profile.vi"("Refnum Name"="STRAIGHT", "Left File Path"=path "/home/lvuser/straight_left.csv", "Right File Path"=path "/home/lvuser/straight_right.csv") -> ()  [unwired: 2 in]
    }
  }
  n116 = global read "CAN.vi" "CAN_ID"() -> (w22:T22)
  n117 = global read "Refnums.vi" "Joysticks"() -> (w26:cluster{"DriverStick":T12, "OperatorStick":T12})
  n118 = Bundle By Name(cluster=w26, "DriverStick"=w24, "OperatorStick"=w14) -> (w23:cluster{"DriverStick":T12, "OperatorStick":T12})
  n119 = global write "Refnums.vi" "Joysticks"(w23) -> ()
  n120 = global write "Robot Global Data.vi" "Robot Mode"(WPI_DriverStationRobotMode2."Autonomous Disabled" ("Robot Mode")) -> ()
  n121 = call-poly <vilib>:"NT Write Value.vi"("String Array"=string[] ["New Name"], "Name"="DB/Button Names") -> ()  [unwired: 9 in, 1 out]
  n122 = call-poly <vilib>:"NT Write Value.vi"("String Array"=string[] ["Alternative 1", "Alternative 2"], "Name"="Auto List") -> ()  [unwired: 9 in, 1 out]
  n123 = global read "Refnums.vi" "Motors"() -> (w21:T23)
  n124 = Bundle By Name(cluster=w21, "ROBOT_DRIVE"=w20, "LEFT_MASTER"=w4, "RIGHT_MASTER"=w3) -> (w17:T23)
  n125 = Bundle By Name(cluster=w17, "AGITATOR OLD"=w5, "AGITATOR"=w6, "INTAKE"=w9, "HOPPER"=w8, "INDEXER"=w7, "TURRET"=w19, "SHOOTER_MASTER"=w16, "SHOOTER_SLAVE"=w10, "SHOOTER_ANGLE"=w13) -> (w18:T23)
  n126 = global write "Refnums.vi" "Motors"(w18) -> ()
  n127 = global read "Refnums.vi" "Pneumatics"() -> (w1:T24)
  n128 = Bundle By Name(cluster=w1, "COMPRESSOR"=w15, "SHIFTER"=w12, "INTAKE_PIVOT"=w11) -> (w2:T24)
  n129 = global write "Refnums.vi" "Pneumatics"(w2) -> ()
  n130 = call "Load Motion Profile.vi"() -> ()  [unwired: 5 in]
  "error out" <- "error in"
